vi "CaenHold.vi"(10 "error in (no error)":errorcluster, 11 "Network Session":refnum<k5>) -> (0 "error out":errorcluster, 1 "PS Response 2":string, 2 "PS Response 1":string, 3 "Network Session Out":refnum<k5>)   [LabVIEW 2025]
doc: "Author: Scott Hannahs <sth@magnet.fsu.edu>\n\nThis software is licensed for use under the “MIT License\"\nCopyright (c) 2025 Scott Hannahs, sth@sth@magnet.sthnet.net\n\nPermission is hereby granted, free of charge, to any person obtaining a copy of this software and associated documentation files (the \"Software\"), to deal in the Software without restriction, including without limitation the rights to use, copy, modify, merge, publish, distribute, sublicense, and/or sell copies of the Software, and to permit persons to whom the Software is furnished to do so, subject to the following conditions: The above copyright notice and this permission notice shall be included in all copies or substantial portions of the Software.\n\nTHE SOFTWARE IS PROVIDED \"AS IS\", WITHOUT WARRANTY OF ANY KIND, EXPRESS OR IMPLIED, INCLUDING BUT NOT LIMITED TO THE WARRANTIES OF MERCHANTABILITY, FITNESS FOR A PARTICULAR PURPOSE AND NONINFRINGEMENT. IN NO EVENT SHALL THE AUTHORS OR COPYRIGHT HOLDERS BE LIABLE FOR ANY CLAIM, DAMAGES OR OTHER LIABILITY, WHETHER IN AN ACTION OF CONTRACT, TORT OR OTHERWISE, ARISING FROM, OUT OF OR IN CONNECTION WITH THE SOFTWARE OR THE USE OR OTHER DEALINGS IN THE SOFTWARE."
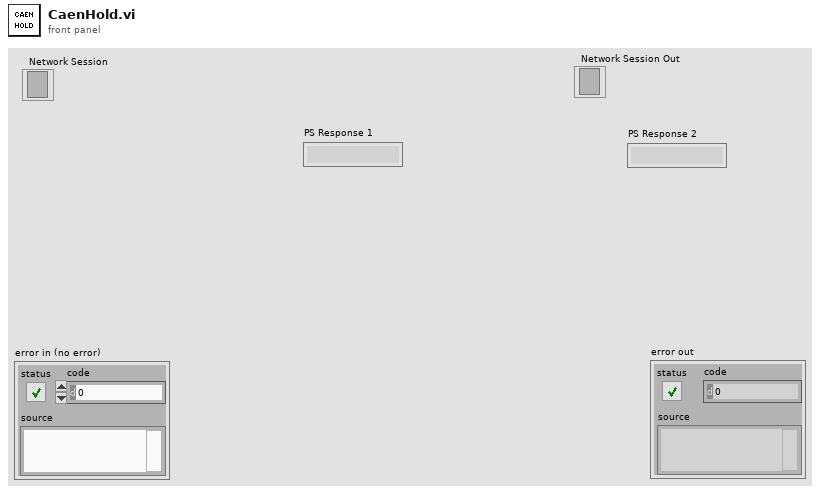
[diagram p1: front panel]
types:
  T1 = enum16{"Standard", "Buffered", "CRLF", "Immediate"}
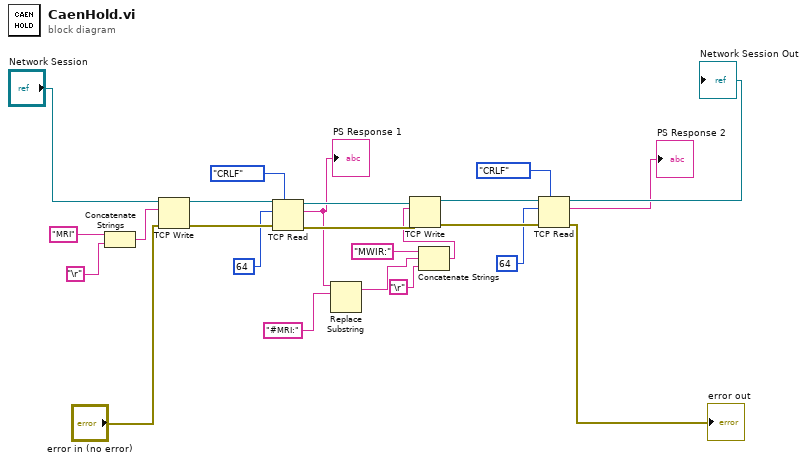
[diagram p0: block diagram]
diagram:
  n1 = Concatenate Strings("MRI", "\r") -> (w17:string)
  n2 = TCP Write(connection ID="Network Session", data in=w17, error in (no error)="error in (no error)") -> (connection ID out=w23:refnum<k5>, error out=w15:errorcluster)  [unwired: 1 in, 1 out]
  n3 = TCP Read(connection ID=w23, bytes to read=64, error in (no error)=w15, 7:T1."CRLF" ("mode (standard)")) -> (connection ID out=w22:refnum<k5>, data out=w9:string, error out=w14:errorcluster)  [unwired: 1 in]
  "PS Response 1" <- w9
  n4 = Replace Substring(4:"#MRI:", 5:w9) -> (1:w5:string)  [unwired: 2 in, 1 out]
  n5 = Concatenate Strings("MWIR:", w5, "\r") -> (w4:string)
  n6 = TCP Write(connection ID=w22, data in=w4, error in (no error)=w14) -> (connection ID out=w21:refnum<k5>, error out=w13:errorcluster)  [unwired: 1 in, 1 out]
  n7 = TCP Read(connection ID=w21, bytes to read=64, error in (no error)=w13, 7:T1."CRLF" ("mode (standard)")) -> (connection ID out=→"Network Session Out":refnum<k5>, data out=→"PS Response 2":string, error out=→"error out":errorcluster)  [unwired: 1 in]
